vi "Set Parameters GUI.vi"(8 "error in (no error)":errorcluster, 11 "Lakeshore 336 in":refnum<class "Lakeshore 336.lvclass">) -> (0 "error out":errorcluster, 3 "Lakeshore 336 out":refnum<class "Lakeshore 336.lvclass">)   [LabVIEW 2022 SP3, in "Lakeshore 336.lvclass"]
uses:
  Lakeshore 336.lvclass
  Lakeshore 336.lvclass/Lakeshore 336.ctl
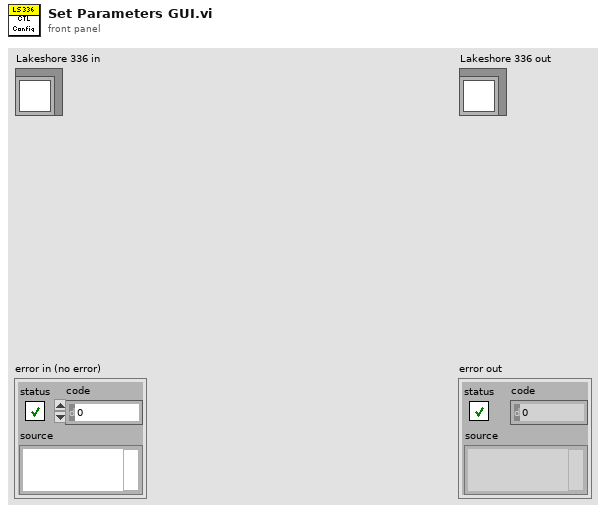
[diagram p1: front panel]
types:
  T1 = typedef "Lakeshore 336.lvclass/Lakeshore 336 Settings cluster.ctl" = cluster{"Lake Shore 336 Address":refnum<visa-resource-name>, "Output Ch":T2[], "Input Ch":T4[], "Prefix":string}
  T2 = typedef "Lakeshore 336.lvclass/Lakeshore 336 Channel Settings cluster.ctl" = cluster{"Input (0:None)":u16, "Power Up Enable (F: Off)":bool, "Mode (0:Off)":u16, "Max Current (0:User Specified)":u16, "Heater Out Display (1:Current)":u16, "Max User Current (2.000)":dbl, "Heater Resistance (1:25 Ohms)":u16, "PID":T3, "Name":string}
  T3 = typedef "Lakeshore 336.lvclass/Lakeshore 336 PID cluster.ctl" = cluster{"P":dbl, "I":dbl, "D":dbl}
  T4 = typedef "Lakeshore 336.lvclass/Lakeshore 336 Input Ch config cluster.ctl" = cluster{"Name":string}
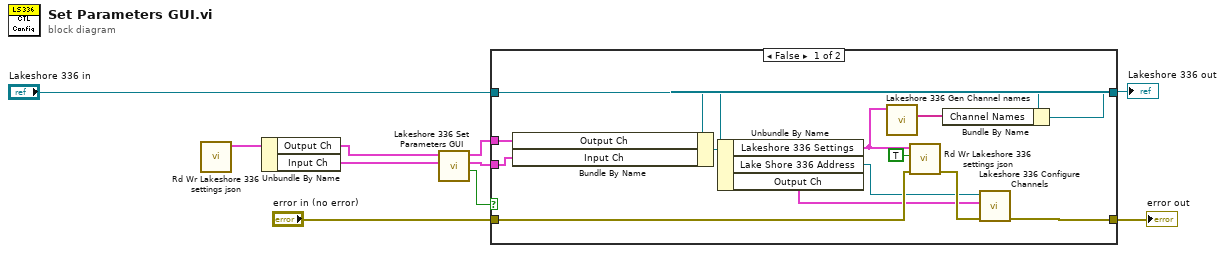
[diagram p0: block diagram]
diagram:
  n1 = call "Rd Wr Lakeshore 336 settings json.vi"() -> ("Lakeshore 336 Settings"=w3:T1)  [unwired: 10 in, 1 out]
  n2 = Unbundle By Name(w3) -> ("Output Ch"=w2:T2[], "Input Ch"=w1:T4[])
  n3 = call "Lakeshore 336 Set Parameters GUI.vi"("Lakeshore 336 Settings.Input Ch"=w1, "Lakeshore 336 Settings.Output Ch"=w2) -> ("Cancelled"=w10:bool, "Lakeshore 336 Settings.Input Ch out"=w6:T4[], "Lakeshore 336 Settings.Output Ch"=w7:T2[])  [unwired: 7 in]
  n4 = case shown="False" w10 {
    tunnel: "Lakeshore 336 in" -> [w21 w24]
    tunnel: [w15 w24] -> w8
    tunnel: w7 -> [w23 _]
    tunnel: w6 -> [w22 _]
    tunnel: "error in (no error)" -> [w19 w25]
    tunnel: [w13 w25] -> w4
    frame False {
      n5 = Bundle By Name(cluster=w21, "Output Ch"=w23, "Input Ch"=w22) -> (w17:refnum<class "Lakeshore 336.lvclass">)
      n6 = Unbundle By Name(w17) -> ("Lakeshore 336 Settings"=w18:T1, "Lake Shore 336 Address"=w12:refnum<visa-resource-name>, "Output Ch"=w11:T2[])
      n7 = call "Lakeshore 336 Gen Channel names.vi"("Lakeshore 336 Settings"=w18) -> ("Channel Names"=w16:string[])  [unwired: 9 in, 1 out]
      n8 = call "Rd Wr Lakeshore 336 settings json.vi"("error in (no error)"=w19, "Write? (F:Read)"=TRUE, "Lakeshore 336 Settings"=w18) -> ("error out"=w14:errorcluster)  [unwired: 7 in, 1 out]
      n9 = Bundle By Name(cluster=w17, "Channel Names"=w16) -> (w15:refnum<class "Lakeshore 336.lvclass">)
      n10 = call "Lakeshore 336 Configure Channels.vi"("error in"=w14, "Ch Setup"=w11, "VISA resource name"=w12) -> ("error out"=w13:errorcluster)  [unwired: 7 in, 1 out]
    }
    frame True {
    }
  }
  "error out" <- w4
  "Lakeshore 336 out" <- w8
